vi "Configure Transient Operation.vi"(0 "VISA resource name":refnum<visa-resource-name>, 1 "Transient Mode (0:Continuous)":u16(ring) items=["Continuous", "Pulse", "Toggle"], 2 "Transient Type (0:CC)":u16(ring) items=["CC", "CV", "CR", "CW"], 5 "A Level Value (1)":dbl=1.0 min=0.0 max=7500.0 step=1.0 format="%.3f", 7 "A Width (1)":dbl=1.0 min=0.0 max=120.0 step=1.0 format="%#.3f", 9 "B Level Value (2)":dbl=2.0 min=0.0 max=7500.0 step=1.0 format="%.3f", 11 "error in (no error)":errorcluster, 12 "B Width (1)":dbl=1.0 min=0.0 max=120.0 step=1.0 format="%#.3f") -> (4 "VISA resource name out":refnum<visa-resource-name>, 15 "error out":errorcluster)   [LabVIEW 2018, in "BK Precision 8600 Series.lvlib"]
doc: "Configures the transient load operation between A level and B level.\n\nNote: The operation mode must be configured first before running this vi. For example, if the transient type is for current (CC mode), configure the load to CC mode using <b>Configure Operation Mode.vi</b> first."
uses:
  <instrlib>/BK Precision 8600 Series/BK Precision 8600 Series.lvlib
panel:
  # "s"
  # "s"
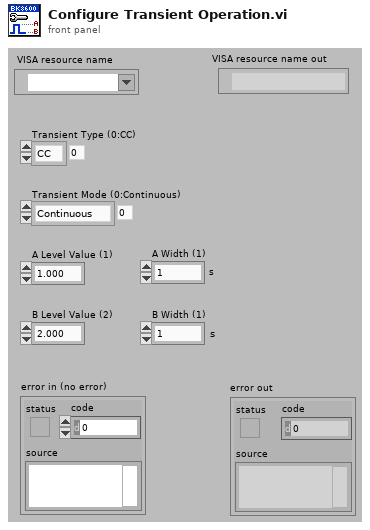
[diagram p1: front panel]
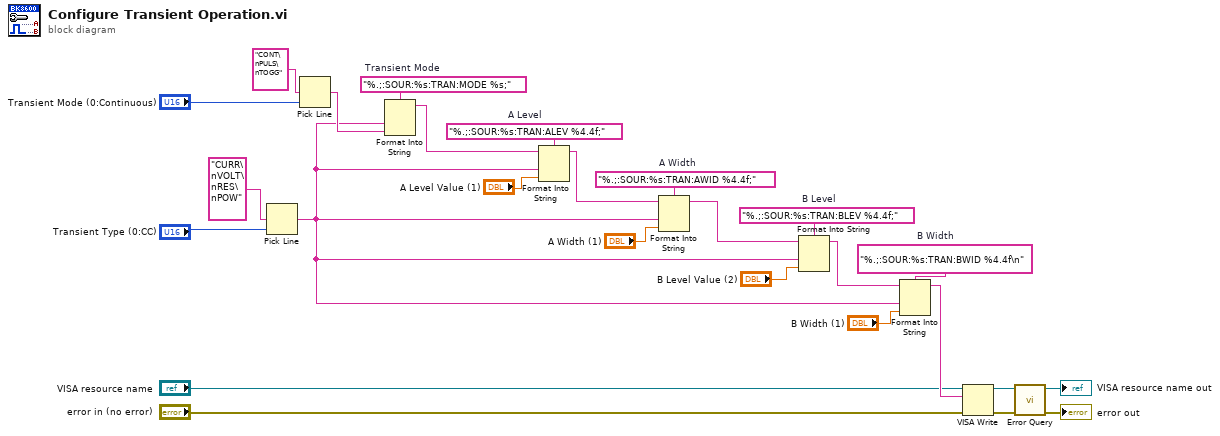
[diagram p0: block diagram]
diagram:
  w18 = "%.;:SOUR:%s:TRAN:BWID %4.4f\n"  # B Width
  w19 = "%.;:SOUR:%s:TRAN:BLEV %4.4f;"  # B Level
  w20 = "%.;:SOUR:%s:TRAN:AWID %4.4f;"  # A Width
  w21 = "%.;:SOUR:%s:TRAN:ALEV %4.4f;"  # A Level
  w22 = "%.;:SOUR:%s:TRAN:MODE %s;"  # Transient Mode
  n1 = Pick Line(multi-line string="CURR\nVOLT\nRES\nPOW", line index="Transient Type (0:CC)") -> (output string=w5:string)  [unwired: 1 in]
  n2 = Pick Line(multi-line string="CONT\nPULS\nTOGG", line index="Transient Mode (0:Continuous)") -> (output string=w6:string)  [unwired: 1 in]
  n3 = Format Into String(format string=w22, w5, w6) -> (resulting string=w16:string)  [unwired: 2 in, 1 out]
  n4 = Format Into String(format string=w21, initial string=w16, w5, "A Level Value (1)") -> (resulting string=w15:string)  [unwired: 1 in, 1 out]
  n5 = Format Into String(format string=w20, initial string=w15, w5, "A Width (1)") -> (resulting string=w14:string)  [unwired: 1 in, 1 out]
  n6 = Format Into String(format string=w19, initial string=w14, w5, "B Level Value (2)") -> (resulting string=w13:string)  [unwired: 1 in, 1 out]
  n7 = Format Into String(format string=w18, initial string=w13, w5, "B Width (1)") -> (resulting string=w12:string)  [unwired: 1 in, 1 out]
  n8 = VISA Write(VISA resource name="VISA resource name", write buffer=w12, error in (no error)="error in (no error)") -> (VISA resource name out=w23:refnum<visa-resource-name>, error out=w24:errorcluster)  [unwired: 1 out]
  n9 = call <instrlib>:"Error Query.vi"("error in (no error)"=w24, "VISA resource name"=w23) -> ("error out"=→"error out":errorcluster, "VISA resource name out"=→"VISA resource name out":refnum<visa-resource-name>)  [unwired: 6 in, 2 out]
